vi "Part 2.vi"(11 "Input":string="^^<<v<<v><v^^<><>^^<v<v^>>^^^><^>v^>v><><><<vv^^<^>^^<v^>v>v^v>>>^<>v<^<v^><^>>>>><<v>>^>>^>v^>><<^>v>v<>^v^v^vvv><>^^>v><v<><>^><^^<vv^v<v>^v>>^v^>v><>v^<vv>^><<v^>vv^<<>v>>><<<>>^<vv<^<>^^vv>>>^><<<<vv^v^>>><><^>v<>^>v<v^v<^vv><^v^><<<<>^<>v>^v>v<v<v<<>v<^<<<v>>>>>^^v>vv^^<>^<>^^^^<^^^v<v^^>v<^^v^^>v>^v^^^^>><<v<>v<>^v^<v<>><>^^><<^^<^^>vv<>v^<^v<vv<<<>^>^^>^<>v^^vv<>>v><<<>vvv<>v<>><^<^v<>^vv>^^v<v<v><^<>>vv<^>>^>>vv^v<vv^vv<^<<>>^v^<>^>>>>vv>^^>v>vv>v><^vv^<<v>^<<^^<v<v>vv<v^^<>^^v>^>>v><^<<vv<<v^vv^^^v>>v<<v^><vv^><vv<^vv<<vv^v<<^v<^^v>><<v^>>^^<>v>><<v<>>^^<v>>^^>>vvv^><<<<<^<^vv<^<><v<<>^^^<<<^>^^^<v<<vv>vv<>^<>v<^v>^<<<v<v<v>>^v<>>v<<^<<v<<>^<<<><><>^>>>>^>v^v<<v<v<<>>vv<^vvv^^^^<vv>vv>^v^^v^<v^v><^vv<^vv>v<^>vv<>>^>^><vv<><^>v>^v>vvv<>^>^v<><>vv>><^v^<><><v>>v^v^><^<^>vv>v<^>vvv>v<<<<<^<v<<vv<^^^<<>>^v<vv<^<>v>^<v<>><><>^<<v>v^>^<vv>><><>>^>^>><^<v>^^>^^>^^v^^<^v^^>v^^>>><<><v<v<<v^vv<><><>^<v>^<<^^v^>v>><>^^^><^vvv<^^^^^v><<><v<^^v><><>>^>vv<vvvv<<>>><v<^^^^v<<^><v>^vv<v^^v^vv<^^>^^<v>><<v^>v<^^>^<^<v<^^v>^<<v>^>>>^v<>v<^^^>vvv^v<<^><>>><vvv^<^^^<^>>v>>><v>^^vvv^vvv<^^^^v^v^<vv^<v>^<<^>v^v^<<><>><^v><v<><<>><<<>^v>v<>^<v^v>^vv>>^<>v^^<<v><^v>>v<>>^v^^>><^>v^<^v^^>><>v^>^v^v<<<v^<v^^v<^>v<><>vv>>>>^>v<>v<<<>^^>vv^v<><v^<>^<<<<>>^^>^v<v^v<<><>^v<>>^v^<<^<^>>>^vv<><v<^^<>v^>>v<^^v<v>>>^>><<><<<>><vv<v>>^v>><^<v><vv>^vv<v<>>><>v^><>vv<^^v^^^v<>><^vvv<<^<>v>>>v>><v><>>><>><v^><v^v<v>^v>v<v>>^^<^>^>v><>vv>^v><<>>>>>>>^<<^vv^^vvvv<^^><<<v<<>vvv<>^><<v<v^v^<<v>v<>>^<vv^<v<v>^<<^^vv>v>^<vv<<>v<v^<>v>>^v^^vvvv>^^>>v^v^^><<^>v>>^^>^<^^<>v<v>vv^vv>v<v>>^v<><^vv^<vv<v^^^v<^v^>>^v>>>^^<^<^>^v^>^>>>^v>^>^^^>>^<>v^^<>^v<<^^>^^<vv<>v<^v^>><^v^>^<>>^vv^vv^>v^<vvvvvv^>><^^<^v<^<v^<<^^<<v^<^>><>v><^v^v^^^v>v^<>^<<v<^^vvv<v>^^>^v^^<><vv^v^>v^<<>>vv<>>>>v>v<>^>>>v<>^^><v<v^^^<>^<^><>^><<v>><>^<<>>><<^<vvv<^><v>>^vv^v>><v<>vv^<<^^<<><v><<^<v<vv<<^v^vv>v^>>>v<<<<v<<>v>^vv<^v><v<v>v<^>^^vv>v><v>><<v<<v^v>>><>^<>><><<^<<^v^v<<v>v>v<v<^^>vv<^v^^^<v^<<<v<>v^><^v>^<^<v>>^<<<v>>v^<><>>^v<>vvv<vvvvv<^^><^>><^^>^>^v^vv<^><<^v>><^^v>^v<>^>vvvv><^>^<<v^^vv<v^^<><>v>^>>^<^<<<^v^^^>^>>^>><><<^>v^^<v>>v<<<<vvv<vvvv^<^<v^^<>^>vvv^<vv^v^v>^<<><v><^v^v^^^>^^>^vv<>v>>v^>vv^vv>v<^v^^>>^v^v<>>^^><<v<<>><>>>^>^<>^^v^^><^<>><<^<vv^^^^^>>vv^<v^<^>>>>v<<><<^>vv>vvv>^<><>>>>vv><<v^v<^^^<<^^^vv^<v<><><<<<>><<v^<>v>v^><>v^v^^><>v>v>^^v<^v<>>^^^^^<v>><v^>^^<v>><v^^>v<^<^>>>^><^^>><<>>^><>^^^>v^^^>^^v^<>^^><^>>><><^>>v<v^>v<^><v<v^<>v<^v>v^<^vv^^><<<><><^v^<v<^^>v>v^>>^^vv^<v>^v>^<^v<>^>^><^<v>^v><^<^<>v^^>^><>>><<v><<><>v<<^v^^<^><>^<><><v>v<^^<v<v>>^^<<>>^<v>><^><^<^>^^v<>v>>><><<>^>v><><<<<v^^^^v<>>^^^v>><<^v>^>>><vv^>>^vv<^<>>^<^^<^v>v<v<<<<<>^<<^<<<<<^<^>>^><<>><>v^v>^<^>v^<><vvv^>^v^v^v><^<v<>vv<<^<>^^^<>^v>^<v^^<v^v>v<>>^>v<<>v<>v^v>v<<<>>v>vv>>v<<>v<>v<^>^>^<v>>v>^>^^^<vv>v<<>>><v>^vvv^^>^^<^vv^^^^>v>^v^>v^^v^>>^v>^vv>^^v^<<<<>^<><^<^<<^^>v^^^v<>>vvv<v>>vv><v<v>^<^v>>^v<vv^<<v<vv><^^v^v>v<>^v<<<^^v^^^<^v>v^v^v>><vvv<<>v<>^v>vv^v>vv<<^v<v>^v>v>><^v<v<>v>>>><<<><vv><>^v^<^vvv>v<>><^v>^>><v>vv<><><>v><>>><^>vv>>^<>v^>>^><<<^><<>^v^>>><><>vv>^<>^>^v^^><^>>><<>v^<^vv>^<^vv>><v<>vv<v><><<^><>v<^^<^>vv^^^^vv<<v><>vv<><v>v<>>>>^><v><>^<><>v<>><<>^^vvv>^^^<><>>vvv^v>><>vv<vv>^^^v^<<>^^v<><<^^v<>^^>^<^^v>>v^v^^>>v>>>^<<^<>^>^^v>>>><vv<<>^v<<vv><<^^vv><^>vv<>>v<v>v^>v>>v^<vv<<<v><v^>vvv^^>vv^<<v>v^>>v^<>>><><<^^<^v>^>>>v>v>^v<>vv><vv<vvv<<v>v>^v<<<>><<><><>v^>>>v^>v^>>vv^^<v>^<>>><^>v^<>^^><v>v<><<<><v^v<<<v<v^>v^v>^>v<^<>v>v^^>>v>vv^v<>>^^^^<>v^>>>>>>>><v<^<<vvv<^v^>^v<^<<>>><<<^<<^>^>v^<>^<<<>v>><^vv^>^>^>>>^<vv><v^^^<v^<v<><v^vvv<>v<vvv^vv<<<v^<^<^vvvv^<<vv<^v><<>^>^<v^v^<^>v^><>>v^>v^>^>>v<>vv^v<<>^^>>vv<>vv>>^v<^vv>^v>v<v^vvv^<<^><>v^<><vv><>v^^><<<><>^>^v^<>><vv<^>v^v>v<>><v<<^>^<vv<^v>^<<v><^<^^vv^<>><v^>^vv^<>>^^^^v>v><^^^v^<<<>^<^<<>><>>v<<^v^>><><v^>>^vv^v>vv>>>>>>^^<<>v^>v^v>^^>>><vv^^^v>^v>>^^^<>><>v^<<<v<vv^^<v^<<<>v>v^^^<vv<>>^v>^v<^<<><>vv>^^^<^^vv<v<<vv>^^>vv>v<<^>^vv><^><v>^^^^v<<vv>v^<<^^>>^^vvvv^v^>vv>>v^<v>vvv<>>^><>>v^^>>^<>>vvvv^>><v^v<^^<^vv>>v<<^<<^><v^^><v^>v^>><<<v>v>v^>^v<v^vv<^^^v<^<vvvvv<<vvv>><>v<v<v<<^v<><<>vv>><v>><^>>^^v>^>><>vv^><<>>vv<<<^<^^>^<<^>>>><v<^v<<<>>v>vv<^>^v><>>v<v^v<>v^vvvv>v^>>v><<^<v>^^v>>vv^^>v>^v>^v^^>^<^vv<v<<^>vv<<^>>^<<^^>>^<^>v^><^vv>^^v><v^>>><>v^v>^v<^><<<>vv><v>v<><>>v^<>^^>^<>^<<^>>vv^><^<v<^^vvv>>v^>>v^>v>vv><>>v<^>><<<v<<vv><v<v<v>v<v>vv^vvv^vv^>^>v><vv<v^^<>>>>vv^>^<>v<^>^<^v>vv<^<<>>^<^<vv><^^<>^<<v^v^>v<<><v>v>><^v<<^vvv>v>v<<^^<^^>v<vv<v<v^v>^^^>^>vv<v<<^^v^<v<^>^^^vv>v<>>>vv>><><^><><<<vvv<<^^v^<v^<<^>>vv>vv^v^>>><v><<v^v>>v>>vv>^^vvv^>^^>^>^>^v<<^vv^>vvv^^vv><^>^v^>^><>v<^^vv<v><v^<><^<>><v>^^v^v>v^vv<>><^v>^<^v>^<>^v>>>><<vv^^^vv^>>><vv^v>>v><^v^vv><<^v<<>^^<v><^v>vvv<><^^><<^v><>^<^v<^^<^vvvv^^>>>>vv>v>>>v<v^><<<<v>>v^><v>>vv^v<vv<>vv<>vvv>>>><>>><>^v<v^v><vvv<<v^^v^v<>>><>>^vv<<v<><<vv<v^>^^vv><^v^v<v^vvv^v>v^^^vv>^><^vvv<<>^vvv^<v<v^v>>>>^<<<><<<<<^v<^^>>>>^>^<v^^^v<vvv<vv^<>v<<<^<^>>v^<v><<><<^^vvv^>v<>>^^>v>^v>>v<v><v>>>>^<^<^>v^v<vv<>^>><>^<<^vvv^^<>^<vvv<>v^>^^<<^>^vv><vvv>>v^v^>v><v>^<^^<>^>^>>>^^vvv^<<>v^<<>><>v<^<^>v^>^vv><v<^<<<^v>^>>^<^v^<<<<^v^><v^v>v^><<v<><<v^<<^<<v<<v><v><><^^^^>v>^^<v>>v<vvv<<<>><>>^><<><^<>>^^>vv<^><^v^><vvv>>>vvv<<vv^<^^^<^>^<>>^>>^v^<^^v>^<v<<>^^v<^vv^><vvv>>^v><<^<v^<><><>>^>vv<<>^^^v^^<v<>><>>vv>v^>vvv^^v<vv<^<^>>^>>^>>v^<<<v^>v^<^v^vv^><^<^v<<v<<>v>^v^<<<v^vv<v<<>^^<v>>>^<v<^>^^v<v>>>><vv<^^<<>><<v<v>^^v^>>^^>>^v^<^v>v^v^v^v^>v^vv<><>^^<>^><^^^<<<^<v>v<<>^<^^^^^v^<^<<^^>^vv<>v^>><>>^>v>v<>^>v<v^>>><>^<><v>>>^>^>>v^><v<>v><^vv^>v<<v>v<><<vv<<v>^><^<v^>v<<v^v<<><v><>v<v><>^^<v<>><<>v>vv<<v>^v<v>vv><><>vv^<<>^>^<^>>>^v>v<^v^^^vv<>>>^<<^>>><<^^v^>v^<^v>vvv>v^^vv>^^>>v<>^<<>^<><^^v^>><>^>v>>^^^<<^^v<>^^>^<>^>><^>^vvv><^>^<^>^>>vv<^>>^v>>^<>>^^>>>v^<v>>v<<v<^>>v^^vv>v><^v^^><vv^v<^>v<<>v^^<><>^>vvv><^^^>^v^>v>>^vvv<^vv>^^>^>>v<>><<^v<<v^>^><>vv^<<^^vv><v>>^<^><^<v>^v<v>^<<>^v^^>v^>>^^^<^vv>v^>>>vv<<>v>>>^>v^^<v^v^^v^>>v<v<<v>^<<>>vv<<^v>v<<vv<<^<^v<^<><^^>v>>v>v^>><vv<^v<^>^>>v>^><<^<<>^v<v>>><^^<^<<<v^^>^>vv<<>^<>^<v^<<^v>vv>^^^v<^v><v<<<<<vv>vv>^^^^>v>v><<^<<<^vv><^<<<><v>><v^v>v<<v^^<v^>v>^v^v^<^<^vv>vvv<^^v<>v<<<<>v<v^<vvv^^^<<^<^<<>^<<><<<>v<^>^^v<^^v^>vv>vvv>v><v^^<<>>^><^>>v<<vv>v<<^^^v<<^v^^><><<<><<>v>^<<>v<<<^v>><v^v<^v<v^vv>v>><<^<><^v^^v<v>^>^>vvvv<<><<>>^<vv>^^><v<>v>v<v^^>^><>>><^><<><<<^<>v^><vv^^^^>>^v^>v^<>>v>^^><^<^v^<v^>>v>^vvv<>>v<v^v><>^vvvv<v^<<v^<<^^vv>><<<<<<v><<<v<v^v^^<v^^<>v<<<<^v<<><<v^<^><v<vv<v^v^<v^^vv<v^v<<<>^<<>vv<v<^>^<<><vv<<vv<v<^<^<>><^^<<>>>vv>>>>>>^v<v<>>v^v^^<v^<<<<>><<^v^^^<>^<vv>>>><>v^v^vvv^>>v>><v^v<<<^v>>^^<<^^vv><<<^^^<<<v><^^>>>>vvv^v<^>^^>v<^<><vv<v<>v>>>^vv<<^<v>^v^>^>^v>v>v^v^>v<<v>><>><v^^<<^>>>><<^v^<>^v<vv><>vvv^>v>v<v<v^>^<><><>^>>><v<<<v^vv><>^>^^<<v^>>v^^>^<v>><>><>v^v^^v>>>>vv>>^v<<^v^<>^>v^^>^^<<vvvvvvv>^<v^<<^<<>><<<^^^v^^^^v<^<>v<^^<>vv^^v^<>^<<^>>v>v<<<^^^^vvv^<^<><>v<<v^<^<>>><<><<<v<v<v><vv>^^<vv<<vv<<<v<^>^^vv<v<>><<>>>^v<<>^>>>v^>v>^^<>^<vv<><^>v>^>>>><>^^>v^^v>^vv^^v^><<<>>v<>v<vv<vv^v^v<^v^<^^><<<><vv^^>^<^<<>v>>>>^<<v>v<v>vv<^><^<v><<^>v>>v><<v<<^v^<>>^>>>^v^v>v^^vv^>^<^^>>^><^vv^^vv^<>>^^^^<^^><><v<>>^>>^><vv^>^vvv<^<<v^^<<<>^><>>>^^<><v<v<><<v^^^^^<^<^<<>><<>>>>^<<>>>^<^v^>><<^>>>^<<v>^>><>^<v>^<><v>^v^^vv<><^>vv^^v^<^^^v^vvv^>><>>v<<vv<>>^<^vvv<<^^><vvv^^<v<>vv^^<<>><v>><^^vvv<<<^>^<><^>vv^><^<<>vv<<v>>vv>v>v^<vv><vv><<>^^^^v^^^^<v>^<<^><><^^v^>v>^>><^><<>v^<v>>>^vvv>>^<^<>^^v^vv^^v><<vv^<>>>v<<<>v>^<>v<<>v^>^<<><<><v<v<v<>v^>v<><^^>^<^v^^><^>vv>^>vv<v<^v>vv>^^><<>vv^>^v<<^<<^<<>v<v<^<v>v>>^><v^^v^v>>>><v^v^<<<vv<<^^<>>v^v<^v>v>^^^v<v><v^^^vv<>v^v<^<>v><><v^<>>vv>v><>v>^v<><<<<<<v<>>v^vv<<<<v<<v><^<>^>><>^^vv>^<^<<>vv>>vv<vvv>><><v<>><^<v>^><^<<v>><v><v>^<v>><>v^^^^v<v^^v<>^^vv<>v<>v>^vv^><v^<<^<>^<>^^^>v^>>>v><<^>>v<^v<>^^<v<><v^v<v>v<><v<vv><<>v<^<^>v<>v^>v>^^<<<^^vv^<><<<>>v>^^<>v>>>><v<v<^^^v<v<v^><<>v^v<>v>><<<<v^<><^<<^>^<vvv<v^^v>>v^vv^><^v^^<>^^><<v^>>vv>^<v^vv<^^v<>>vvv<^v^>>^<v<v>>^>^^<<^>^>^v><>>^<^^v>^>>^^<><>>>^^>^^vvv>v<^^<>v^v^^<v<<^<v^v^<<>v^v<v<<v<>>><<^^^>>v>^vv>^>^^v<>^^<>v^^<><v<v<vvv^<vv<<>v^><<><v<>vv<<^vvvv><<<v>v>v^>v^<>v^>^<v<vvv^>^<>^>^^v<>><<<><v<^^>^v<v>^^v^v<<<^v^<>^<>v>^^>v<v<v>v>^^<<<><<^>v<v<^vv^v><^^<<vv>^<<v><>^>>>>><v^v<<<^>^v^v<<v<>vvv<<>v>v>>^v^v^>><<<<>v^<v<><<>>>^>>^>><<v>") -> (3 "Output":i64)   [LabVIEW 2021]
uses:
  ab2fd95b-bc5c-494e-9d3b-f0a391d2a47b.vi
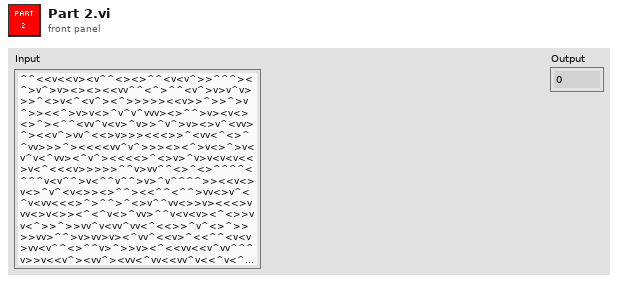
[diagram p1: front panel]
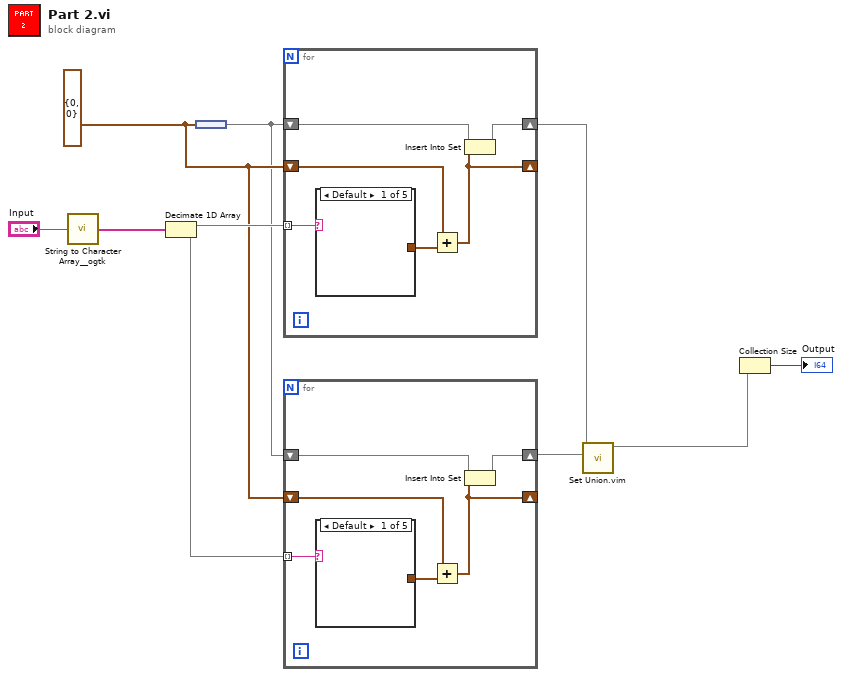
[diagram p0: block diagram]
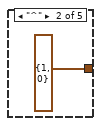
[diagram p2: hidden frame]
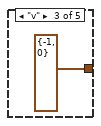
[diagram p3: hidden frame]
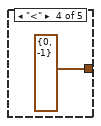
[diagram p4: hidden frame]
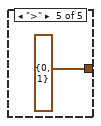
[diagram p5: hidden frame]
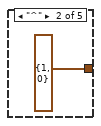
[diagram p6: hidden frame]
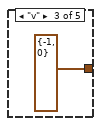
[diagram p7: hidden frame]
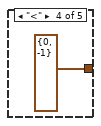
[diagram p8: hidden frame]
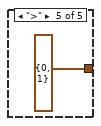
[diagram p9: hidden frame]
diagram:
  w5 = cluster{"X":i32, "Y":i32} {"X"=0, "Y"=0}
  n1 = call <userlib>:"String to Character Array__ogtk.vi"("Input String"="Input") -> ("Character Array"=w9:string[])
  n2 = Decimate 1D Array(w9) -> (w7:string[], w6:string[])
  n3 = node(w5) -> (w4:set{cluster{"X":i32, "Y":i32}})
  n4 = for {
    tunnel: w7 -> [w16] mode=indexing
    shift-right: [w12] -> w3
    shift-left: w4 -> [w13]
    shift-right: [w11] -> _
    shift-left: w5 -> [w14]
    n5 = case shown="Default" w16 {
      tunnel: [_ cluster{"X":i32, "Y":i32} {"X"=1, "Y"=0} cluster{"X":i32, "Y":i32} {"X"=-1, "Y"=0} cluster{"X":i32, "Y":i32} {"X"=0, "Y"=-1} cluster{"X":i32, "Y":i32} {"X"=0, "Y"=1}] -> w15
      frame Default {
      }
      frame "^" {
      }
      frame "v" {
      }
      frame "<" {
      }
      frame ">" {
      }
    }
    n6 = Add(x=w14, y=w15) -> (x+y=w11:cluster{"X":i32, "Y":i32})
    n7 = Insert Into Set(10:w11, 11:w13) -> (3:w12:set{cluster{"X":i32, "Y":i32}})  [unwired: 1 out]
  }
  n8 = for {
    tunnel: w6 -> [w26] mode=indexing
    shift-right: [w22] -> w2
    shift-left: w4 -> [w23]
    shift-right: [w21] -> _
    shift-left: w5 -> [w24]
    n9 = case shown="Default" w26 {
      tunnel: [_ cluster{"X":i32, "Y":i32} {"X"=1, "Y"=0} cluster{"X":i32, "Y":i32} {"X"=-1, "Y"=0} cluster{"X":i32, "Y":i32} {"X"=0, "Y"=-1} cluster{"X":i32, "Y":i32} {"X"=0, "Y"=1}] -> w25
      frame Default {
      }
      frame "^" {
      }
      frame "v" {
      }
      frame "<" {
      }
      frame ">" {
      }
    }
    n10 = Add(x=w24, y=w25) -> (x+y=w21:cluster{"X":i32, "Y":i32})
    n11 = Insert Into Set(10:w21, 11:w23) -> (3:w22:set{cluster{"X":i32, "Y":i32}})  [unwired: 1 out]
  }
  n12 = call "Set Union.vim"("set 2"=w2, "set 1"=w3) -> ("union"=w1:set{cluster{"X":i32, "Y":i32}})  [unwired: 9 in]
  n13 = Collection Size(1:w1) -> (0:→"Output":i32)
